vi "motor_control.vi"() -> ()   [LabVIEW 2014]
uses:
  <vilib>/Platform/TimedLoop/XDataNode/timing_clust.ctl
  <vilib>/Platform/TimedLoop/XDataNode/nitl_modes.ctl
  <vilib>/Platform/TimedLoop/XDataNode/wakeup.ctl
  <vilib>/myRIO/Instrument Drivers/Onboard IO/PWM/vis/Set Duty Cycle and Frequency.vi
  <vilib>/myRIO/Instrument Drivers/Onboard IO/DIO/vis/Write.vi
  <vilib>/myRIO/Instrument Drivers/Onboard IO/Encoder/vis/Read.vi
  <vilib>/myRIO/Instrument Drivers/Onboard IO/PWM/vis/Smart Open.vi
  <vilib>/Utility/error.llb/Error Cluster From Error Code.vi
  <vilib>/myRIO/Common/Instrument Driver Framework/myRIO v1.0/PWM/vis/myRIO v1.0 Write PWM.vi
  <vilib>/myRIO/Instrument Drivers/Onboard IO/DIO/vis/Smart Open.vi
  <vilib>/myRIO/Common/Instrument Driver Framework/myRIO v1.0/DIO/vis/myRIO v1.0 Write DIO.vi
  <vilib>/myRIO/Instrument Drivers/Onboard IO/Encoder/vis/Smart Open.vi
  <vilib>/myRIO/Common/Instrument Driver Framework/myRIO v1.0/Encoder/vis/myRIO v1.0 Read Encoder.vi
  <vilib>/platform/TimedLoop/XDataNode/XDataNode.xnode
  <vilib>/Platform/TimedLoop/XDataNode/XDNodeRunTimeDep.lvlib
panel:
  out "position_B":i32
  in  "Reset_B":bool
  out "velocity_B":dbl(graph)
  out "velocity_A":dbl(graph)
  in  "Reset_A":bool
  out "position_A":i32
  in  "电机开关":bool
  in  "B_Duty":dbl(slide) scale=-1.0..1.0
  in  "关闭程序":bool
  in  "A_Duty":dbl(slide) scale=-1.0..1.0
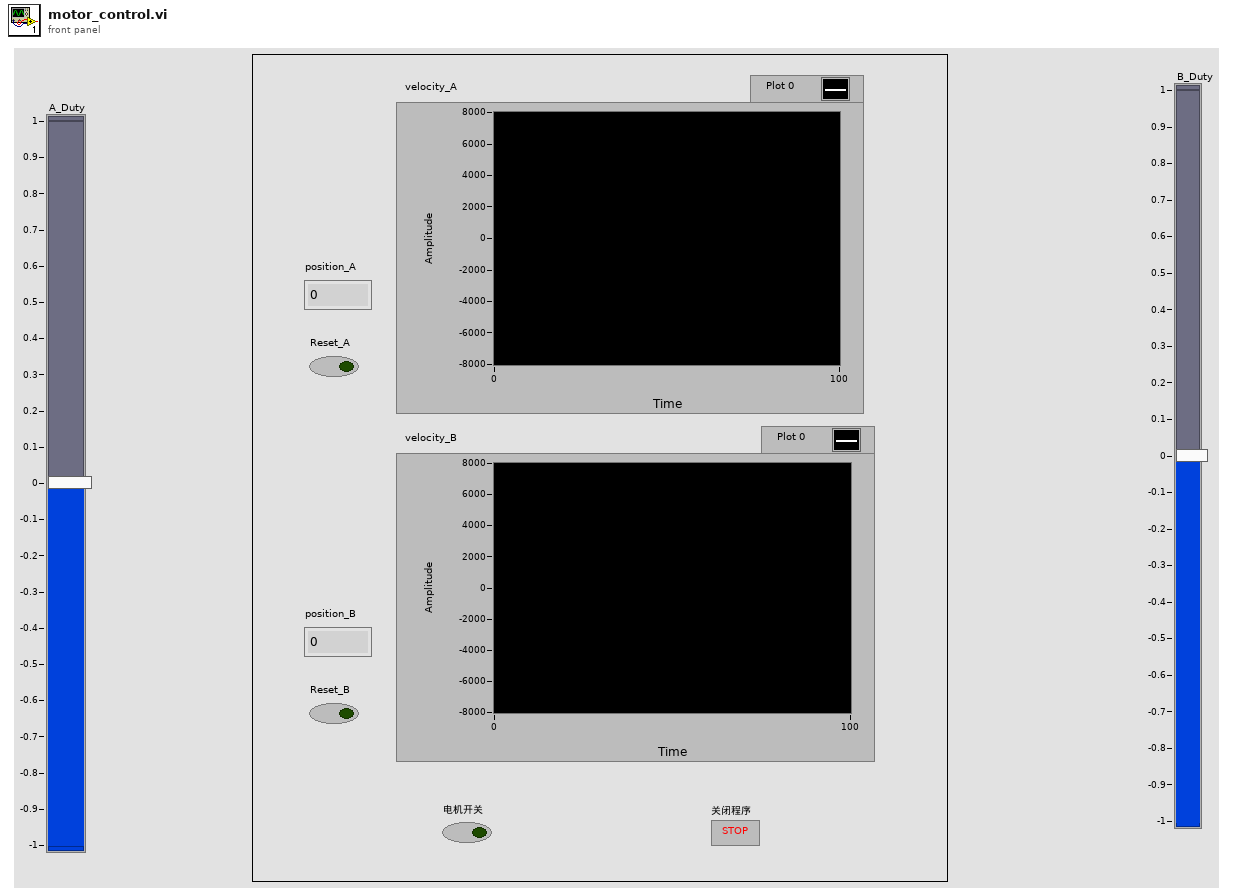
[diagram p1: front panel]
types:
  T1 = typedef "XDNodeRunTimeDep.lvlib/timing_clust.ctl" = cluster{"Expected End [f-1]":u64, "Actual End [f-1]":u64, "Finished Late? [f-1]":bool, "Expected End [i-1]":u64, "Actual End [i-1]":u64, "Finished Late? [i-1]":bool, "Expected Start [i]":u64, "Actual Start [i]":u64, "Expected Start [f]":u64, "Actual Start [f]":u64, "Source Name":string, "Structure Name":string, "Period":i64, "Deadline":i64, "Offset":i64, "Start":i64, "Priority":i32, "Timeout":i32, "Mode":T2, "Wakeup Reason":T3, "Error":errorcluster, "Source Type":string, "Secondary Source Type":string, "Global End Time":u64, "Global Start Time":u64, "Frame Duration":u64, "Iteration Duration":u64, "Assigned CPU":i32, "I/O Scan Engine Mode":u32}
  T2 = typedef "XDNodeRunTimeDep.lvlib/nitl_modes.ctl" = enum32{"No Change", "Process missed periods, maintain original phase", "Discard missed periods, maintain original phase", "Process missed periods, ignore original phase", "Discard missed periods, ignore original phase"}
  T3 = typedef "XDNodeRunTimeDep.lvlib/wakeup.ctl" = enum32{"Normal", "Aborted", "Asynchronous wakeup", "Timing source error", "Timed loop error", "Timeout"}
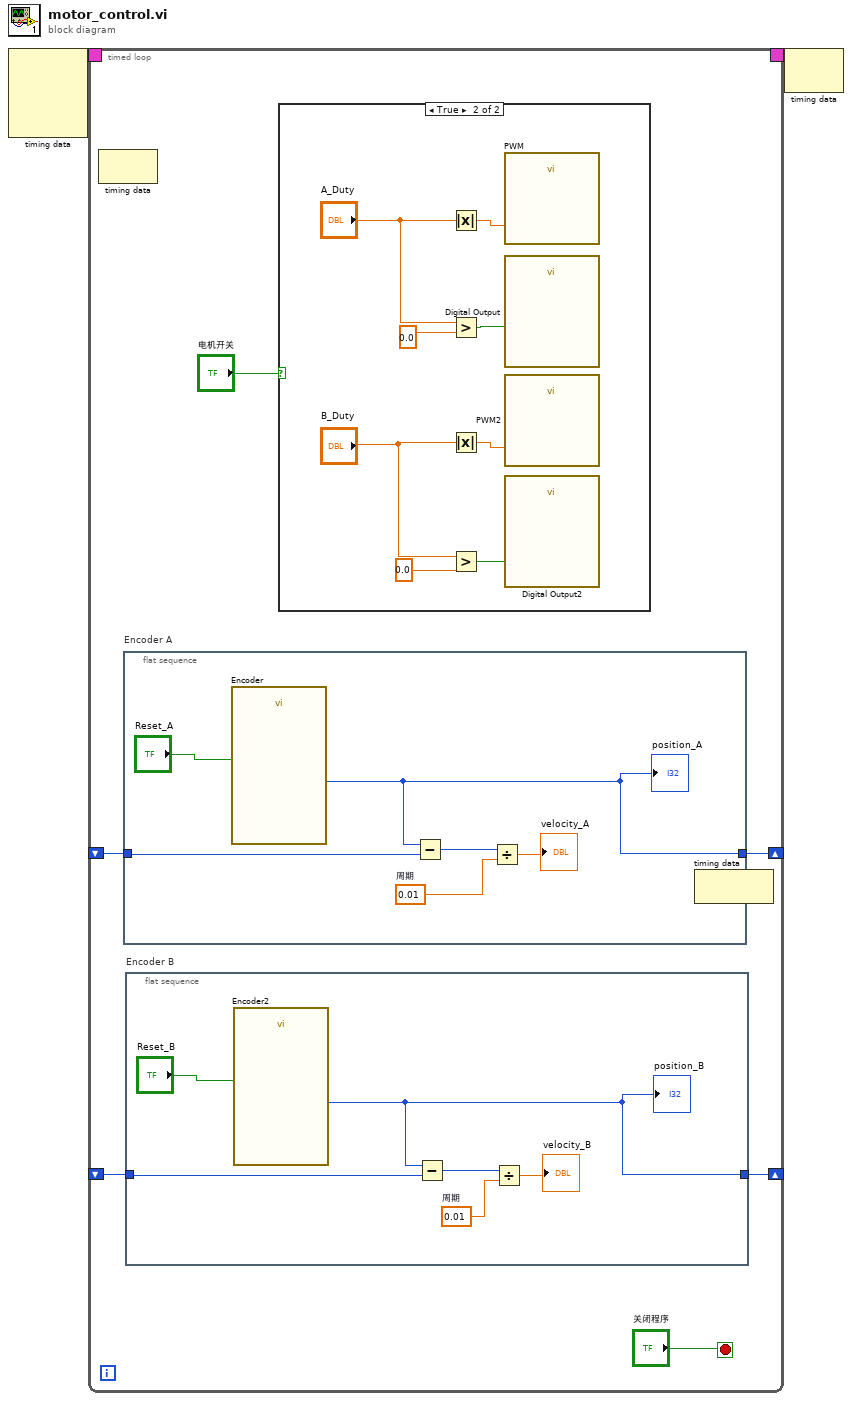
[diagram p0: block diagram]
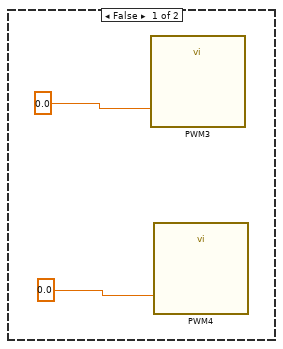
[diagram p2: hidden frame]
diagram:
  n1 = node-c288() -> (w2:T1)  [unwired: 4 in]
  n2 = timed-loop {
    timing: w2 -> [_]
    timing-out: [_] -> w1
    shift-right: [w6] -> _
    shift-left: _ -> [w5]
    shift-right: [w3] -> _
    shift-left: _ -> [w4]
    stop <- "关闭程序" stop-if-true
    n3 = node-c288() -> ()  [unwired: 1 in, 1 out]
    n4 = flat-sequence "Encoder A" {
      tunnel: [w19] -> w6
      tunnel: w5 -> [w18]
      frame #0 {
        w16 = 0.01  # 周期
        n5 = call "Encoder"("Reset Counter"="Reset_A") -> ("Counter Value"=w19:i32)  [unwired: 23 in, 3 out]
        "position_A" <- w19
        n6 = Subtract(x=w19, y=w18) -> (x-y=w17:i32)
        n7 = Divide(x=w17, y=w16) -> (x/y=→"velocity_A":dbl)
      }
    }
    n8 = flat-sequence "Encoder B" {
      tunnel: [w13] -> w3
      tunnel: w4 -> [w12]
      frame #0 {
        w10 = 0.01  # 周期
        n9 = call "Encoder2"("Reset Counter"="Reset_B") -> ("Counter Value"=w13:i32)  [unwired: 23 in, 3 out]
        "position_B" <- w13
        n10 = Subtract(x=w13, y=w12) -> (x-y=w11:i32)
        n11 = Divide(x=w11, y=w10) -> (x/y=→"velocity_B":dbl)
      }
    }
    n12 = case shown="True" "电机开关" {
      frame False {
        n13 = call "PWM3"("Duty Cycle (0-1)"=0.0) -> ()  [unwired: 26 in, 1 out]
        n14 = call "PWM4"("Duty Cycle (0-1)"=0.0) -> ()  [unwired: 26 in, 1 out]
      }
      frame True {
        n15 = Absolute Value(x="A_Duty") -> (abs(x)=w28:dbl)
        n16 = Greater?(x="A_Duty", y=0.0) -> (0:w29:bool)
        n17 = Absolute Value(x="B_Duty") -> (abs(x)=w24:dbl)
        n18 = Greater?(x="B_Duty", y=0.0) -> (0:w23:bool)
        n19 = call "PWM"("Duty Cycle (0-1)"=w28) -> ()  [unwired: 26 in, 1 out]
        n20 = call "Digital Output"("A/DIO0 (Pin 11)"=w29) -> ()  [unwired: 26 in, 1 out]
        n21 = call "PWM2"("Duty Cycle (0-1)"=w24) -> ()  [unwired: 26 in, 1 out]
        n22 = call "Digital Output2"("B/DIO0 (Pin 11)"=w23) -> ()  [unwired: 26 in, 1 out]
      }
    }
    n23 = node-c288() -> ()  [unwired: 1 in, 1 out]
  }
  n24 = node-c288(w1) -> ()  [unwired: 1 out]
